vi "playing with luanching with system exec not use.vi"() -> ()   [LabVIEW 2020]
panel:
  out "standard error":string
  out "standard output":string
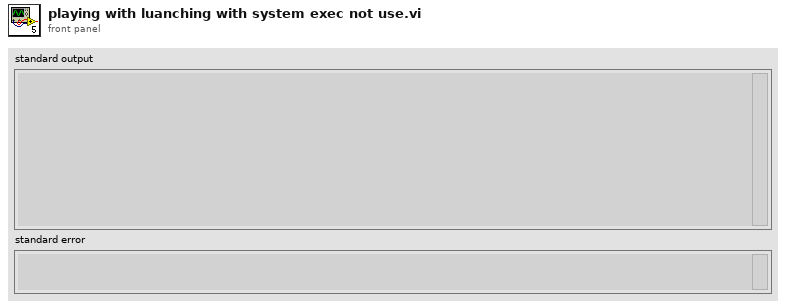
[diagram p1: front panel]
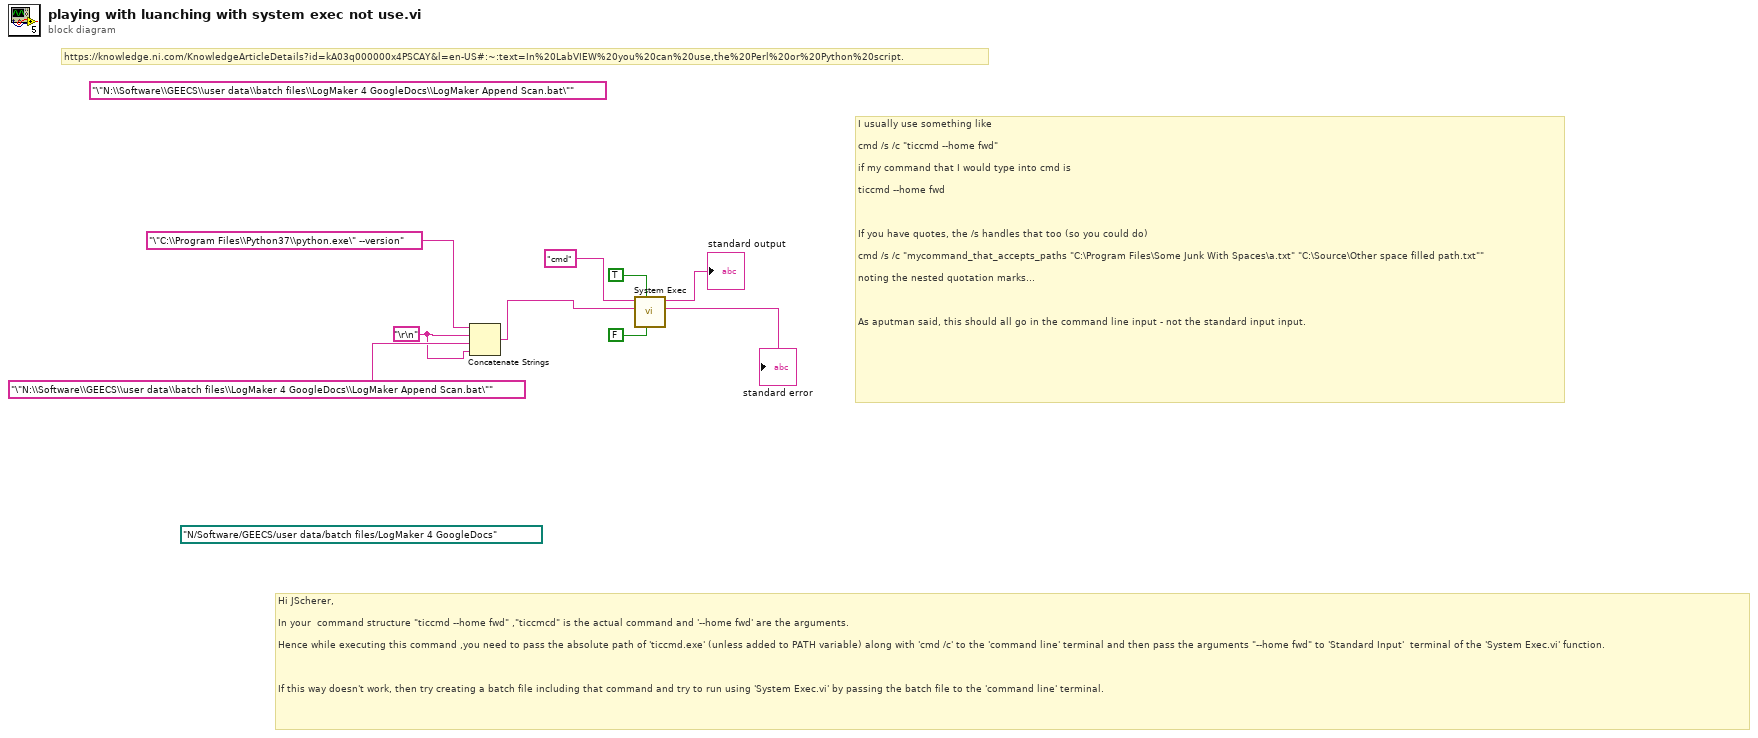
[diagram p0: block diagram]
diagram:
  (unwired) "\"N:\\Software\\GEECS\\user data\\batch files\\LogMaker 4 GoogleDocs\\LogMaker Append Scan.bat\"" ("standard input")
  (unwired) path "N:/Software/GEECS/user data/batch files/LogMaker 4 GoogleDocs" ("working directory")
  w1 = "\r\n"
  # "https://knowledge.ni.com/KnowledgeArticleDetails?id=kA03q000000x4PSCAY&l=en-US#:~:text=In%20LabVIEW%20you%20can%20use,the%20Perl%20or%20Python%20script."
  # "Hi JScherer,\n\nIn your  command structure \"ticcmd --home fwd\" ,\"ticcmcd\" is the actual command and '--home fwd' are the arguments.\n\nHence while executing this command ,you need to pass the absolute path of 'ticcmd.exe' (unless added to PATH variable) along with 'cmd /c' to the 'command line' terminal and then pass the arguments \"--home fwd\" to 'Standard Input'  terminal of the 'System Exec.vi' function.\n\n \n\nIf this way doesn't work, then try creating a batch file including that command and try to run using 'System Exec.vi' by passing the batch file to the 'command line' terminal."
  # "I usually use something like \n\ncmd /s /c \"ticcmd --home fwd\"\n\nif my command that I would type into cmd is\n\nticcmd --home fwd\n\n \n\nIf you have quotes, the /s handles that too (so you could do)\n\ncmd /s /c \"mycommand_that_accepts_paths \"C:\\Program Files\\Some Junk With Spaces\\a.txt\" \"C:\\Source\\Other space filled path.txt\"\"\n\nnoting the nested quotation marks...\n\n \n\nAs aputman said, this should all go in the command line input - not the standard input input."
  n1 = Concatenate Strings("\"C:\\Program Files\\Python37\\python.exe\" --version" ("standard input"), w1, "\"N:\\Software\\GEECS\\user data\\batch files\\LogMaker 4 GoogleDocs\\LogMaker Append Scan.bat\"" ("string"), w1) -> (w4:string)
  n2 = call <vilib>:"System Exec.vi"("run minimized? (F)"=FALSE, "wait until completion? (T)"=TRUE, "standard input"=w4, "command line"="cmd" ("Scan states")) -> ("standard error"=→"standard error":string, "standard output"=→"standard output":string)  [unwired: 4 in, 2 out]
